vi "Init_Test.vi"(8 "error in (no error)":errorcluster caption="entrée d'erreur (pas d'erreur)", 11 "Get_Voltage en entrée":refnum<class "Disable_Relay.lvclass">) -> (0 "error out":errorcluster caption="sortie d'erreur", 3 "Get_Voltage en sortie":refnum<class "Disable_Relay.lvclass">)   [LabVIEW 2020, in "Library Test.lvlib" / "Disable_Relay.lvclass"]
uses:
  Disable_Relay.lvclass
  C:/Users/ngarcin/OneDrive - Altyor/Standard TB/Class/Test/Test (Default)/Test (Default).lvclass
  Commun VI/TypeDef/Commande Test/Commande Value Type.ctl
  Commun VI/TypeDef/Commande Test/Commande Type Test.ctl
  Commun VI/TypeDef/Commande Relay_Board/Data_Write_Relay_Board.ctl
  Commun VI/TypeDef/Commande Relay_Board/Parameter Relay_Board.ctl
  Relay_Board/Relay_Board (Default)/Class Relay_Board (Default).lvclass
  JSON API/JSON Value/Set from JSON string.vi
  JSON API/Variant JSON/Variant to JSON.vi
  JSON API/JSON Value/Get Item by name array.vi
  Test_Wtih_Instr/Test_With_Inst.lvclass
  Instrument/Instrument (Default)/Class Instrument (Default).lvclass
  JSON API/JSON Value/JSON Value.lvclass
  Disable_Relay.lvclass/Disable_Relay.ctl
  JSON API/Get Polymorphic/JSON GetSet.lvlib
  JSON API/Variant JSON/Variant JSON.lvlib
  Commun VI/Library Commun.lvlib
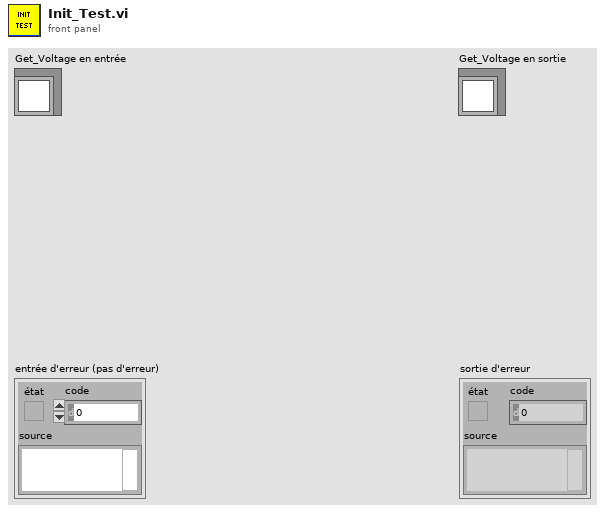
[diagram p1: front panel]
types:
  T1 = typedef "Library Commun.lvlib/Commande Type Test.ctl" = enum16{"Function", "Test", "Calculation"}
  T2 = typedef "Library Commun.lvlib/Commande Value Type.ctl" = enum16{"None", "String", "Number", "Timestamp", "Boolean", "Array"}
  T3 = typedef "Library Commun.lvlib/Data_Write_Relay_Board.ctl" = enum16{"Enable Relays", "Disable Relays"}
  T4 = typedef "Library Commun.lvlib/Parameter Relay_Board.ctl" = cluster{"Device_Com_Port":string, "Address Board":string, "Tab_Num_Relay":u8[], "Parameter Class Relay_Board":refnum<class "Class Relay_Board (Default).lvclass">}
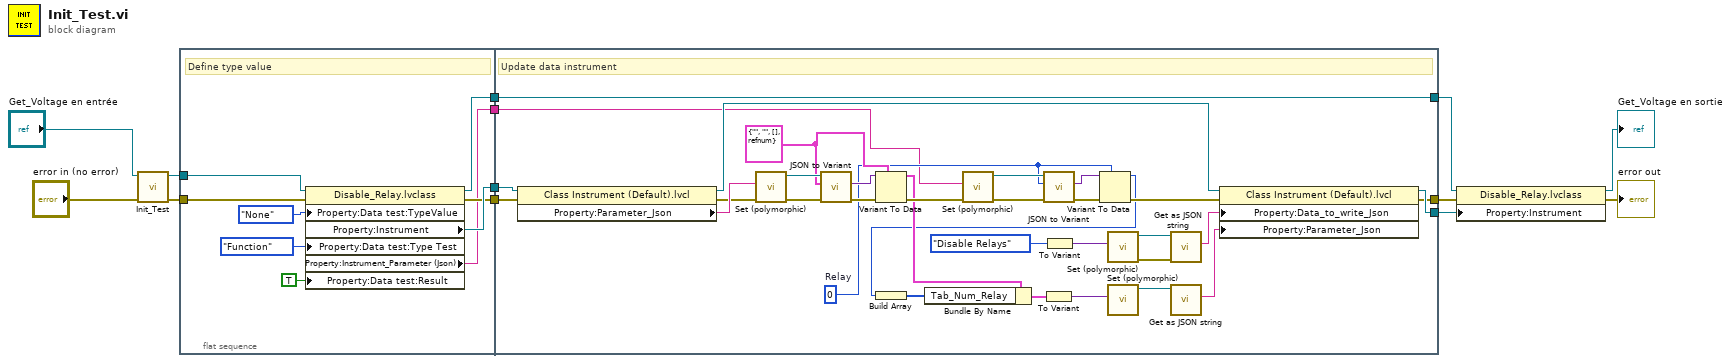
[diagram p0: block diagram]
diagram:
  n1 = call-parent "Init_Test.vi"("error in (no error)"="error in (no error)", "Test_With_Inst en entrée"="Get_Voltage en entrée") -> ("error out"=w10:errorcluster, "Test_With_Inst en sortie"=w11:refnum<class "Disable_Relay.lvclass">)  [unwired: 8 in]
  n2 = flat-sequence {
    tunnel: w11 -> [w22]
    tunnel: w10 -> [w21]
    tunnel: [w20] -> w4
    tunnel: [w17] -> w3
    tunnel: [w16] -> w2
    tunnel: [w15] -> w1
    tunnel: [w26] -> w7
    tunnel: [w28] -> w8
    tunnel: [w25] -> w9
    tunnel: w4 -> [w29]
    tunnel: w3 -> [w27]
    tunnel: w2 -> [w25]
    tunnel: w1 -> [w24]
    frame #0 {
      # "Define type value"
      n3 = property class="Disable_Relay.lvclass"(reference=w22, error in=w21, "Property:Data test:TypeValue"=Commande_Value_Type."None" ("TypeValue"), "Property:Data test:Type Test"=Commande_Type_Test."Function" ("Type Test"), "Property:Data test:Result"=TRUE ("Result")) -> (reference out=w16:refnum<class "Disable_Relay.lvclass">, error out=w17:errorcluster, "Property:Instrument"=w20:refnum<class "Class Instrument (Default).lvclass">, "Property:Instrument_Parameter (Json)"=w15:string)
    }
    frame #1 {
      w37 = T4 {"Device_Com_Port"="", "Address Board"="", "Tab_Num_Relay"=[], "Parameter Class Relay_Board"=refnum} ("Parameter")
      w36 = 0  # Relay
      # "Update data instrument"
      n4 = property class="Class Instrument (Default).lvcl"(reference=w29, error in=w27) -> (reference out=w30:refnum<class "Class Instrument (Default).lvclass">, error out=w40:errorcluster, "Property:Parameter_Json"=w42:string)
      n5 = call-poly "Set (polymorphic).vi"("error in (no error)"=w40, "JSON stream"=w42) -> ("error out"=w44:errorcluster, "JSON Value out"=w46:refnum<class "JSON Value.lvclass">)  [unwired: 7 in, 1 out]
      n6 = call "JSON to Variant.vi"("error in (no error)"=w44, "Variant (Data Type)"=w37, "JSON Value"=w46) -> ("error out"=w45:errorcluster, "Variant out"=w43:variant)  [unwired: 7 in]
      n7 = Variant To Data(error in=w45, type=w37, Variant=w43) -> (data=w38:T4, error out=w41:errorcluster)
      n8 = call-poly "Set (polymorphic).vi"("error in (no error)"=w41, "JSON stream"=w24) -> ("error out"=w49:errorcluster, "JSON Value out"=w47:refnum<class "JSON Value.lvclass">)  [unwired: 7 in, 1 out]
      n9 = call "JSON to Variant.vi"("error in (no error)"=w49, "Variant (Data Type)"=w36, "JSON Value"=w47) -> ("error out"=w48:errorcluster, "Variant out"=w50:variant)  [unwired: 7 in]
      n10 = To Variant(anything=Data_Write_Relay_Board."Disable Relays" ("Function")) -> (Variant=w55:variant)
      n11 = Variant To Data(error in=w48, type=w36, Variant=w50) -> (data=w23:i32, error out=w39:errorcluster)
      n12 = Build Array(w23) -> (w35:i32[])
      n13 = Bundle By Name(cluster=w38, "Tab_Num_Relay"=w35) -> (w33:T4)
      n14 = To Variant(anything=w33) -> (Variant=w32:variant)
      n15 = call-poly "Set (polymorphic).vi"("Variant"=w55) -> ("error out"=w53:errorcluster, "JSON Value out"=w54:refnum<class "JSON Value.lvclass">)  [unwired: 9 in]
      n16 = call-poly "Set (polymorphic).vi"("Variant"=w32) -> ("JSON Value out"=w34:refnum<class "JSON Value.lvclass">)  [unwired: 9 in, 1 out]
      n17 = call "Get as JSON string.vi"("error in (no error)"=w53, "JSON Value in"=w54) -> ("<JSON>"=w52:string)  [unwired: 8 in, 1 out]
      n18 = call "Get as JSON string.vi"("JSON Value in"=w34) -> ("<JSON>"=w31:string)  [unwired: 9 in, 1 out]
      n19 = property class="Class Instrument (Default).lvcl"(reference=w30, error in=w39, "Property:Data_to_write_Json"=w52, "Property:Parameter_Json"=w31) -> (reference out=w28:refnum<class "Class Instrument (Default).lvclass">, error out=w26:errorcluster)
    }
  }
  n20 = property class="Disable_Relay.lvclass"(reference=w9, error in=w7, "Property:Instrument"=w8) -> (reference out=→"Get_Voltage en sortie":refnum<class "Disable_Relay.lvclass">, error out=→"error out":errorcluster)
